vi "CursorMoveSet.vi"(7 "Enum":T1(ring)=enum."ScrollRight", 8 "错误输入":errorcluster caption="错误输入（无错误）", 11 "WG":refnum<vi>) -> (0 "错误输出":errorcluster)   [LabVIEW 2012]
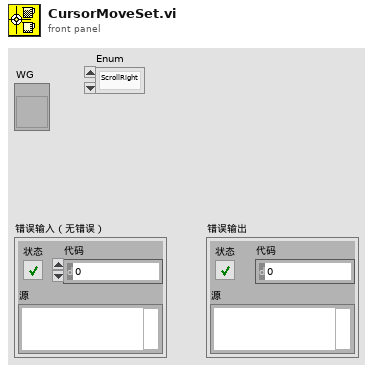
[diagram p1: front panel]
types:
  T1 = enum16{"JumpLeft", "JumpRight", "ScrollLeft", "ScrollRight"}
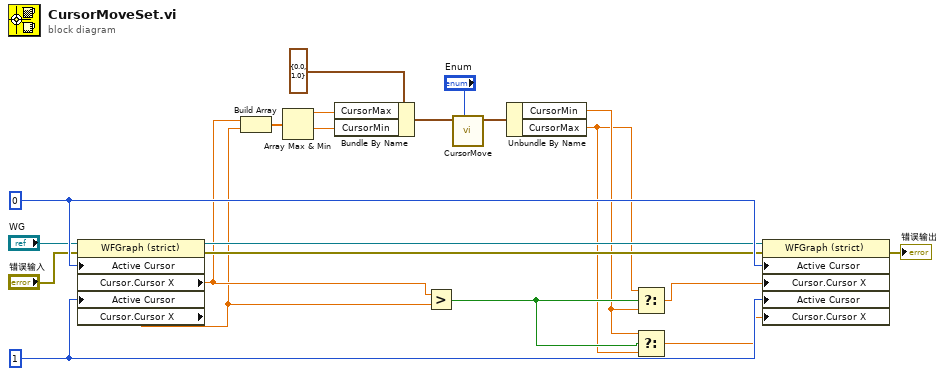
[diagram p0: block diagram]
diagram:
  w21 = u32 1 ("活动游标")
  w20 = u32 0 ("活动游标")
  n1 = property on="属性节点" class="WFGraph (strict)"(reference="WG", error in="错误输入", "Active Cursor"=w20, "Active Cursor"=w21) -> (reference out=w10:refnum<vi>, error out=w9:errorcluster, "Cursor.Cursor X"=w7:dbl, "Cursor.Cursor X"=w6:dbl)
  n2 = Build Array(w7, w6) -> (w19:dbl[])
  n3 = Array Max & Min(array=w19) -> (max value=w13:dbl, min value=w12:dbl)  [unwired: 2 out]
  n4 = Bundle By Name(cluster=cluster{"CursorMin":dbl, "CursorMax":dbl} {"CursorMin"=0.0, "CursorMax"=1.0} ("Cursor"), "CursorMax"=w13, "CursorMin"=w12) -> (w11:cluster{"CursorMin":dbl, "CursorMax":dbl})
  n5 = Greater?(x=w7, y=w6) -> (0:w4:bool)
  n6 = call "CursorMove.vi"("Enum"="Enum", "Cursor"=w11) -> ("Cursor"=w8:cluster{"CursorMin":dbl, "CursorMax":dbl})  [unwired: 9 in]
  n7 = Unbundle By Name(w8) -> ("CursorMin"=w3:dbl, "CursorMax"=w2:dbl)
  n8 = Select(t=w2, s=w4, f=w3) -> (s? t:f=w5:dbl)
  n9 = Select(t=w3, s=w4, f=w2) -> (s? t:f=w1:dbl)
  n10 = property on="属性节点" class="WFGraph (strict)"(reference=w10, error in=w9, "Active Cursor"=w20, "Cursor.Cursor X"=w5, "Active Cursor"=w21, "Cursor.Cursor X"=w1) -> (error out=→"错误输出":errorcluster)  [unwired: 1 out]
